vi "Get Next.vi"(0 "Conditional in":refnum<class "Conditional.lvclass">, 1 "Linked List Ref":refnum<data-value>, 5 "Active Unique ID":string, 9 "Active Element Index":i32, 11 "error in (no error)":errorcluster) -> (3 "Linked List Ref out":refnum<data-value>, 4 "Executioner out":refnum<class "Executioner.lvclass">, 6 "Active Unique ID out":string, 8 "Test Executive Ref out":refnum<data-value>, 10 "Active Element Index out":i32, 12 "Found":bool, 13 "Complete":bool, 14 "Stop":bool, 15 "error out":errorcluster)   [LabVIEW 2020, in "Test Executive.lvlib" / "Conditional.lvclass"]
uses:
  <vilib>/gpm_packages/@cs/test-executive/Source/Test Executive/Conditional/Conditional.lvclass
  C:/Program Files/National Instruments/LabVIEW 2020/vi.lib/gpm_packages/@cs/test-executive/Source/Test Executive/Executioner/Executioner.lvclass
  <vilib>/gpm_packages/@cs/test-executive/Source/Test Executive/Executioner/Executioner.lvclass
  <vilib>/gpm_packages/@cs/linked-list/Source/Linked List/ILinkedList/ILinked List.lvclass
  <vilib>/gpm_packages/@cs/test-executive/Source/Test Executive/ITestExecutive/ITest Executive.lvclass
  <vilib>/gpm_packages/@cs/run-time-assertions/Source/Assert/Assert.lvclass
  28516125-fb7c-4ac0-a741-55c0088c8a73.vi
  9cce5d6f-acb7-42fe-8a76-34eb137fd1f1.vi
  ae19bcc6-c34a-426c-aaf2-8c0212fd8e02.vi
  24807a66-3041-465e-b619-213d0f35a6f1.vi
  60ecfbe6-bfaf-4739-a238-c250300aa515.vi
  e5c56d01-fc27-46d4-835c-91294360ed0c.vi
  8776d587-be4e-442f-99b1-068521ee802a.vi
  8afe6501-fe05-4816-a73f-941b7a14c2e9.vi
  0ff8ee5d-2cdd-4139-ab50-0f64d05a4c29.vi
  ded76606-da74-46a9-a0bc-d95ca2e54d8f.vi
  <vilib>/gpm_packages/@cs/linked-list/Source/Linked List/Linked List Ref/Linked List Ref.lvclass
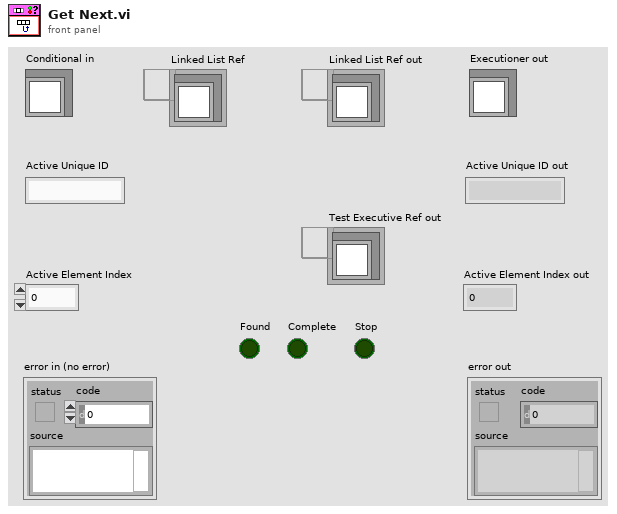
[diagram p1: front panel]
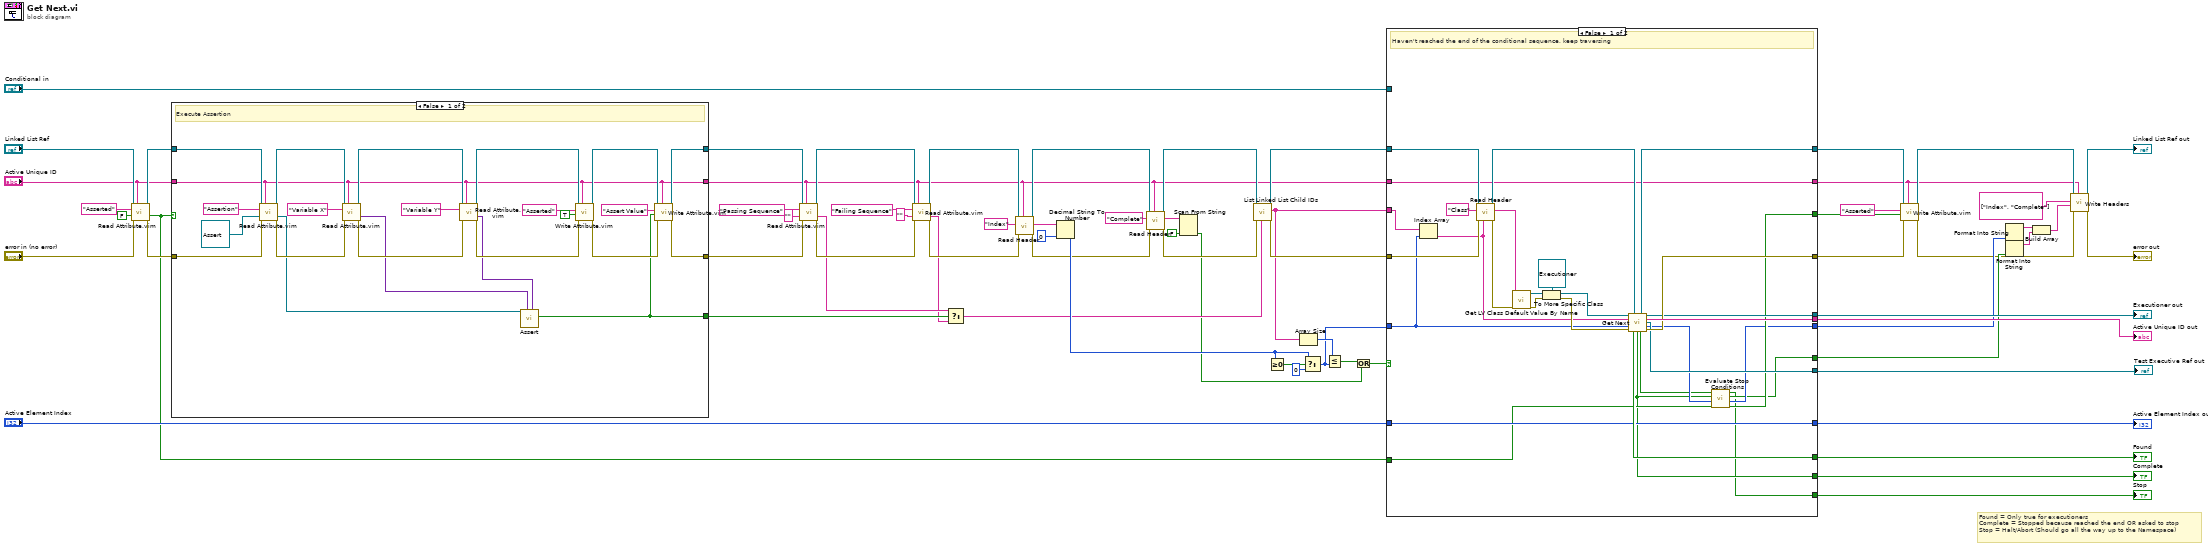
[diagram p0: block diagram]
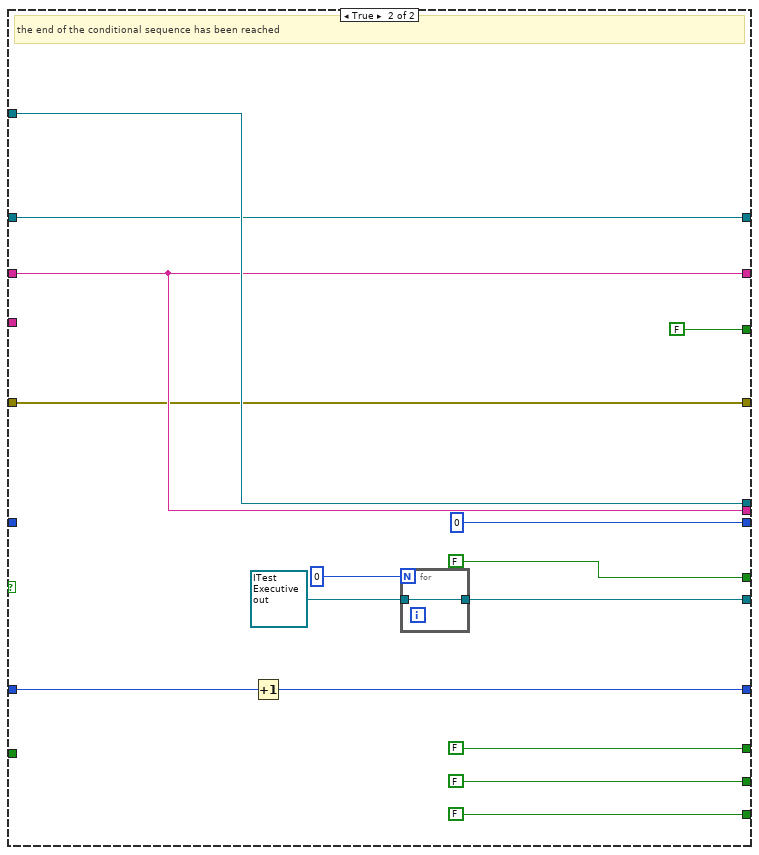
[diagram p2: hidden frame]
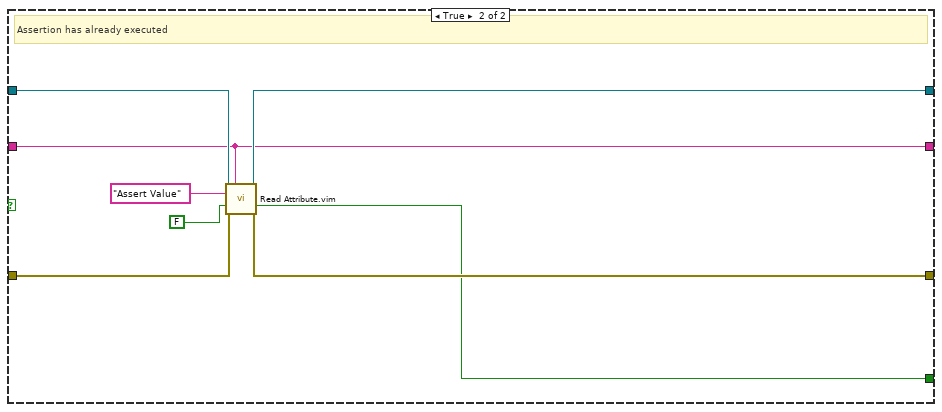
[diagram p3: hidden frame]
diagram:
  # "Found = Only true for executioners\nComplete = Stopped because reached the end OR asked to stop\nStop = Halt/Abort (Should go all the way up to the Namespace)"
  n1 = call "Read Attribute.vim"("Linked List Ref"="Linked List Ref", "Linked List ID"="Active Unique ID", "Attribute Name"="Asserted", "Type"=FALSE, "error in (no error)"="error in (no error)") -> ("Linked List Ref out"=w66:refnum<data-value>, "Attribute"=w1:bool, "error out"=w64:errorcluster)  [unwired: 5 in, 3 out]
  n2 = case shown="False" w1 {
    tunnel: "Active Unique ID" -> [w73 w94]
    tunnel: [w81 w97] -> w61
    tunnel: [w79 w95] -> w62
    tunnel: w66 -> [w86 w98]
    tunnel: w64 -> [w85 w96]
    tunnel: [w69 w93] -> w54
    tunnel: [w73 w94] -> w13
    frame False {
      # "Execute Assertion"
      n3 = call "Read Attribute.vim"("Linked List Ref"=w86, "Linked List ID"=w73, "Attribute Name"="Assertion", "Type"=refnum<class "Assert.lvclass"> refnum ("Run Time Assertions.lvlib:Assert.lvclass"), "error in (no error)"=w85) -> ("Linked List Ref out"=w90:refnum<data-value>, "Attribute"=w70:refnum<class "Assert.lvclass">, "error out"=w89:errorcluster)  [unwired: 5 in, 3 out]
      n4 = call "Read Attribute.vim"("Linked List Ref"=w90, "Linked List ID"=w73, "Attribute Name"="Variable X", "error in (no error)"=w89) -> ("Linked List Ref out"=w76:refnum<data-value>, "Attribute"=w72:variant, "error out"=w77:errorcluster)  [unwired: 6 in, 3 out]
      n5 = call "Read Attribute.vim"("Linked List Ref"=w76, "Linked List ID"=w73, "Attribute Name"="Variable Y", "error in (no error)"=w77) -> ("Linked List Ref out"=w74:refnum<data-value>, "Attribute"=w71:variant, "error out"=w75:errorcluster)  [unwired: 6 in, 3 out]
      n6 = call-dynamic "Assert.vi"("Variable Y"=w71, "Variable X"=w72, "Assert in"=w70) -> ("Assert?"=w69:bool)  [unwired: 8 in]
      n7 = call "Write Attribute.vim"("Linked List ID"=w73, "error in (no error)"=w75, "Attribute"=TRUE, "Attribute Name"="Asserted", "Linked List Ref"=w74) -> ("error out"=w80:errorcluster, "Linked List Ref out"=w82:refnum<data-value>)  [unwired: 3 in, 2 out]
      n8 = call "Write Attribute.vim"("Linked List ID"=w73, "error in (no error)"=w80, "Attribute"=w69, "Attribute Name"="Assert Value", "Linked List Ref"=w82) -> ("error out"=w79:errorcluster, "Linked List Ref out"=w81:refnum<data-value>)  [unwired: 3 in, 2 out]
    }
    frame True {
      # "Assertion has already executed"
      n9 = call "Read Attribute.vim"("Linked List Ref"=w98, "Linked List ID"=w94, "Attribute Name"="Assert Value", "Type"=FALSE, "error in (no error)"=w96) -> ("Linked List Ref out"=w97:refnum<data-value>, "Attribute"=w93:bool, "error out"=w95:errorcluster)  [unwired: 5 in, 3 out]
    }
  }
  n10 = call "Read Attribute.vim"("Linked List Ref"=w61, "Linked List ID"=w13, "Attribute Name"="Passing Sequence", "Type"="", "error in (no error)"=w62) -> ("Linked List Ref out"=w56:refnum<data-value>, "Attribute"=w31:string, "error out"=w55:errorcluster)  [unwired: 5 in, 3 out]
  n11 = call "Read Attribute.vim"("Linked List Ref"=w56, "Linked List ID"=w13, "Attribute Name"="Failing Sequence", "Type"="", "error in (no error)"=w55) -> ("Linked List Ref out"=w53:refnum<data-value>, "Attribute"=w30:string, "error out"=w52:errorcluster)  [unwired: 5 in, 3 out]
  n12 = Select(t=w31, s=w54, f=w30) -> (s? t:f=w29:string)
  n13 = call <vilib>:"Read Header.vi"("Linked List ID"=w13, "error in (no error)"=w52, "Header Name"="Index" ("Attribute Name"), "Linked List Ref"=w53) -> ("error out"=w12:errorcluster, "Header Value"=w26:string, "Linked List Ref out"=w15:refnum<data-value>)  [unwired: 4 in, 1 out]
  n14 = Decimal String To Number(string=w26, default (0L)=0 ("Attribute")) -> (number=w48:i32)  [unwired: 1 in, 1 out]
  n15 = call <vilib>:"Read Header.vi"("Linked List ID"=w13, "error in (no error)"=w12, "Header Name"="Complete" ("Attribute Name"), "Linked List Ref"=w15) -> ("error out"=w11:errorcluster, "Header Value"=w17:string, "Linked List Ref out"=w14:refnum<data-value>)  [unwired: 4 in, 1 out]
  n16 = Scan From String(input string=w17, default 1=FALSE) -> (output 1=w9:bool)  [unwired: 3 in, 3 out]
  n17 = call <vilib>:"List Linked List Child IDs.vi"("Linked List ID"=w29, "error in (no error)"=w11, "Linked List Ref"=w14) -> ("error out"=w46:errorcluster, "Child IDs"=w45:string[], "Linked List Ref out"=w47:refnum<data-value>)  [unwired: 6 in]
  n18 = Greater Or Equal To 0?(x=w48) -> (x >= 0?=w51:bool)
  n19 = Array Size(array=w45) -> (size(s)=w49:i32)
  n20 = Select(t=w48, s=w51, f=0) -> (s? t:f=w44:i32)
  n21 = Less Or Equal?(x=w49, y=w44) -> (x <= y?=w19:bool)
  n22 = Or(x=w19, y=w9) -> (x .or. y?=w10:bool)
  n23 = case shown="False" w10 {
    tunnel: [w121 w133] -> w6
    tunnel: w47 -> [w123 w133]
    tunnel: [w117 w132] -> w4
    tunnel: w46 -> [w125 w132]
    tunnel: w45 -> [w114 _]
    tunnel: w44 -> [w113 _]
    tunnel: [w105 0 ("Active Element Index out")] -> w33
    tunnel: [w109 w142] -> w39
    tunnel: [w120 w138] -> w38
    tunnel: [w119 FALSE ("Found")] -> w43
    tunnel: [w104 FALSE] -> w42
    tunnel: [w101 FALSE] -> w41
    tunnel: "Conditional in" -> [_ w142]
    tunnel: w13 -> [w116 w138]
    tunnel: [w116 w138] -> w3
    tunnel: "Active Element Index" -> [w115 w140]
    tunnel: [w115 w139] -> w36
    tunnel: [w103 FALSE ("Complete")] -> w28
    tunnel: [w111 w134] -> w20
    tunnel: [w107 FALSE] -> w2
    tunnel: w1 -> [w108 _]
    frame False {
      # "Haven't reached the end of the conditional sequence, keep traversing"
      n24 = Index Array(array=w114, index=w113) -> (element=w112:string)
      n25 = call <vilib>:"Read Header.vi"("Linked List ID"=w112, "error in (no error)"=w125, "Header Name"="Class", "Linked List Ref"=w123) -> ("error out"=w118:errorcluster, "Header Value"=w130:string, "Linked List Ref out"=w122:refnum<data-value>)  [unwired: 4 in, 1 out]
      n26 = call <vilib>:"Get LV Class Default Value By Name.vi"("error in (no error)"=w118, "class name"=w130) -> ("error out"=w126:errorcluster, "object"=w129:refnum<class>)  [unwired: 8 in]
      n27 = To More Specific Class(target class=refnum<class "Executioner.lvclass"> refnum ("Test Executive.lvlib:Executioner.lvclass"), reference=w129, error in=w126) -> (specific class reference=w110:refnum<class "Executioner.lvclass">, error out=w127:errorcluster)
      n28 = call-dynamic "Get Next.vi"("Executioner in"=w110, "Linked List Ref"=w122, "Active Unique ID"=w112, "Active Element Index"=w113, "error in (no error)"=w127) -> ("Linked List Ref out"=w121:refnum<data-value>, "Executioner out"=w109:refnum<class "Executioner.lvclass">, "Active Unique ID out"=w120:string, "Test Executive Ref out"=w111:refnum<data-value>, "Active Element Index out"=w106:i32, "Found"=w119:bool, "Complete"=w104:bool, "Stop"=w102:bool, "error out"=w117:errorcluster)  [unwired: 2 in]
      n29 = call <vilib>:"Evaluate Stop Conditions.vi"("Assert"=w108, "Index"=w106, "Complete"=w104, "Stop"=w102) -> ("Asserted"=w107:bool, "Index out"=w105:i32, "Completed"=w103:bool, "Stop out"=w101:bool)  [unwired: 4 in]
    }
    frame True {
      # "the end of the conditional sequence has been reached"
      n30 = Increment(x=w140) -> (x+1=w139:i32)
      n31 = for {
        N: 0 -> [_]
        tunnel: refnum<data-value> refnum ("Test Executive Ref out") -> [w146]
        tunnel: [w146] -> w134
      }
    }
  }
  "Executioner out" <- w39
  "Active Unique ID out" <- w38
  "Active Element Index out" <- w36
  "Found" <- w43
  "Complete" <- w42
  "Stop" <- w41
  "Test Executive Ref out" <- w20
  n32 = call "Write Attribute.vim"("Linked List ID"=w3, "error in (no error)"=w4, "Attribute"=w2, "Attribute Name"="Asserted", "Linked List Ref"=w6) -> ("error out"=w5:errorcluster, "Linked List Ref out"=w7:refnum<data-value>)  [unwired: 3 in, 2 out]
  n33 = Format Into String(w33) -> (resulting string=w23:string)  [unwired: 3 in, 1 out]
  n34 = Format Into String(w28) -> (resulting string=w21:string)  [unwired: 3 in, 1 out]
  n35 = Build Array(w23, w21) -> (w22:string[])
  n36 = call <vilib>:"Write Headers.vi"("Linked List ID"=w3, "error in (no error)"=w5, "Header Values"=w22, "Header Names"=string[] ["Index", "Complete"], "Linked List Ref"=w7) -> ("error out"=→"error out":errorcluster, "Linked List Ref out"=→"Linked List Ref out":refnum<data-value>)  [unwired: 5 in]
